vi "util_createDAQconfig.vi"() -> ()   [LabVIEW 2013]
uses:
  <vilib>/userdefined/High Color/IMAQdx.ctl
panel:
  out "value":cluster{"Sound AO":tag, "Shock intesity AO":tag}
  out "xml string":string
  in  "Master-9 DO":tag="Dev6/port0/line5:7"
  in  "Tone trigger":string="PFI1"
  in  "Sound card":u32
  in  "sample rate":dbl=100000.0 min=8000.0
  in  "Webcam on":bool
  in  "Webcam":T1="cam9"
  in  "Variable shock":bool=TRUE
  in  "AO <=> Sound card":bool
  in  "Shock intesity AO":tag="Dev6/ao1"
  in  "Sound AO":tag="Dev6/ao0"
  in  "Code_LED DO":tag="Dev6/port1:2"
  in  "Switch DI":tag="Dev6/port1/line0"
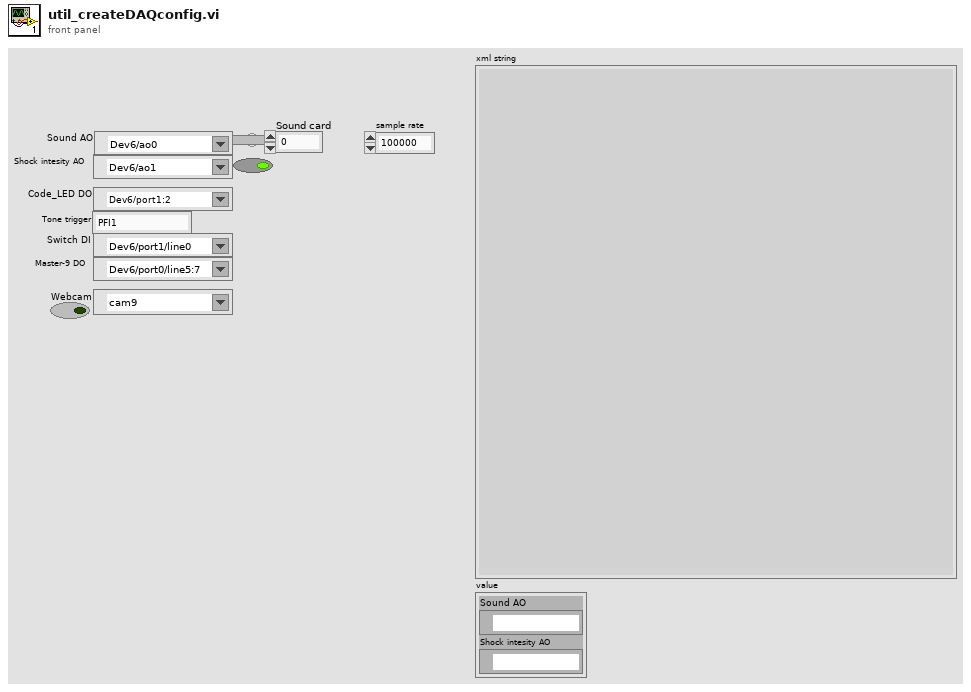
[diagram p1: front panel]
types:
  T1 = typedef "IMAQdx.ctl" = refnum<k21>
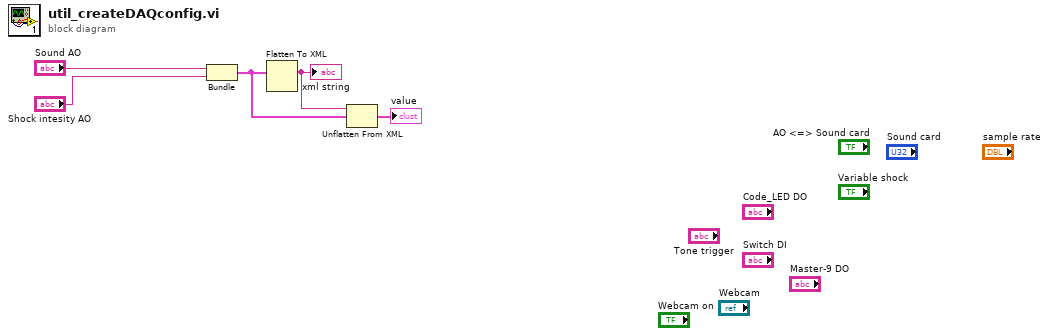
[diagram p0: block diagram]
diagram:
  n1 = Bundle("Sound AO"="Sound AO", "Shock intesity AO"="Shock intesity AO") -> (w2:cluster{"Sound AO":tag, "Shock intesity AO":tag})  [unwired: 1 in]
  n2 = Flatten To XML(anything=w2) -> (xml string=w3:string)
  "xml string" <- w3
  n3 = Unflatten From XML(xml string=w3, type=w2) -> (value=→"value":cluster{"Sound AO":tag, "Shock intesity AO":tag})  [unwired: 1 in, 1 out]
